vi "Write Config.vi"(10 "Config":T1, 11 "Pump_1AI_1DO_2DI in":refnum<class "Valve_2DO_2DI.lvclass">) -> (3 "Pump_1AI_1DO_2DI out":refnum<class "Valve_2DO_2DI.lvclass">)   [LabVIEW 2019, in "Valve_2DO_2DI.lvclass"]
uses:
  Valve_2DO_2DI.lvclass
  Config.ctl
  Valve_2DO_2DI.lvclass/Valve_2DO_2DI.ctl
  TypeDef/bool_setting.ctl
  Sig_DA_class/Sig_DA.lvclass/Sig_DA.ctl
  Sig_DA_class/Sig_DA.lvclass
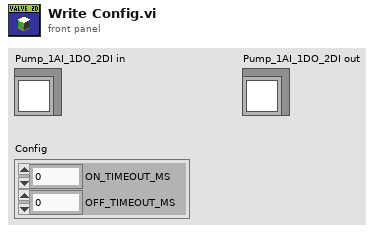
[diagram p1: front panel]
types:
  T1 = typedef "Valve_2DO_2DI.lvclass/Config.ctl" = cluster{"ON_TIMEOUT_MS":dbl, "OFF_TIMEOUT_MS":dbl}
  T2 = typedef "bool_setting.ctl" = cluster{"TON_ms":u32, "TOFF_ms":u32}
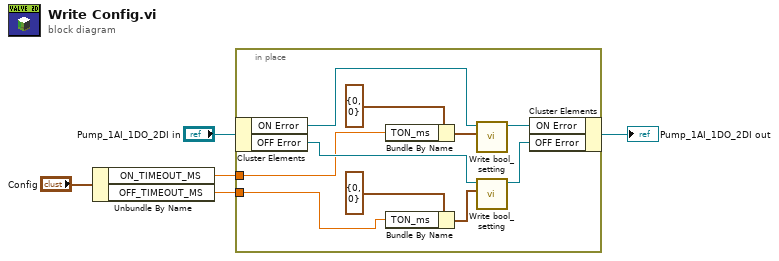
[diagram p0: block diagram]
diagram:
  n1 = Unbundle By Name("Config") -> ("ON_TIMEOUT_MS"=w2:dbl, "OFF_TIMEOUT_MS"=w1:dbl)
  n2 = in-place {
    in-place-border: w2 -> [w8]
    in-place-border: w1 -> [w6]
    n3 = in-place-cluster #1("Pump_1AI_1DO_2DI in") -> ("ON Error"=w15:refnum<class "Sig_DA.lvclass">, "OFF Error"=w13:refnum<class "Sig_DA.lvclass">)
    n4 = Bundle By Name(cluster=T2 {"TON_ms"=0, "TOFF_ms"=0} ("bool_setting"), "TON_ms"=w8) -> (w9:T2)
    n5 = Bundle By Name(cluster=T2 {"TON_ms"=0, "TOFF_ms"=0} ("bool_setting"), "TON_ms"=w6) -> (w7:T2)
    n6 = call "Write bool_setting.vi"("bool_setting"=w9, "Sig_DA in"=w15) -> ("Sig_DA out"=w14:refnum<class "Sig_DA.lvclass">)  [unwired: 9 in]
    n7 = call "Write bool_setting.vi"("bool_setting"=w7, "Sig_DA in"=w13) -> ("Sig_DA out"=w12:refnum<class "Sig_DA.lvclass">)  [unwired: 9 in]
    n8 = in-place-cluster #1("ON Error"=w14, "OFF Error"=w12) -> (→"Pump_1AI_1DO_2DI out":refnum<class "Valve_2DO_2DI.lvclass">)
  }
